vi "WM Create Wave Buffer with Phase Angle.vi"(2 "Buffer Info":T2 {"Paddle Height" format="%.2f"; "Water Depth" format="%.2f"}, 3 "Sine Paramaters":T1 {"Phase Angle (rad)" format="%.2f"; "Wave Height" format="%.2f"; "Period" format="%.2f"}) -> (0 "Output":dbl[](array[numeric]) format="%.2f", 1 "Buffer Size":i32)   [LabVIEW 2012]
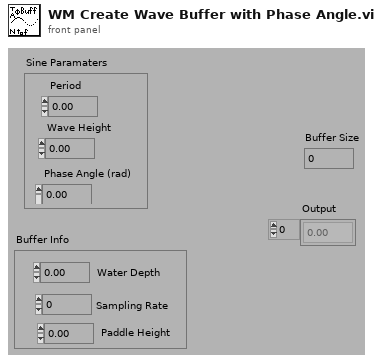
[diagram p1: front panel]
types:
  T1 = cluster{"Period":dbl, "Wave Height":dbl, "Phase Angle (rad)":dbl}
  T2 = cluster{"Sampling Rate":i32, "Water Depth":dbl, "Paddle Height":dbl}
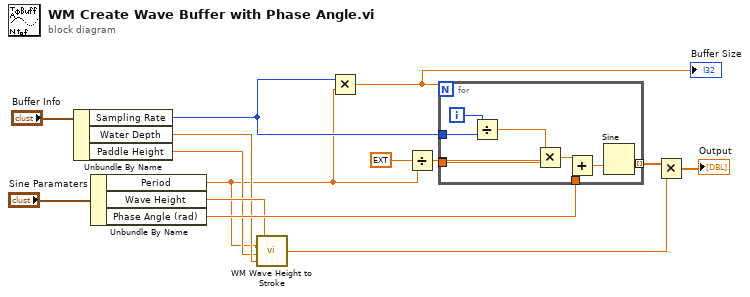
[diagram p0: block diagram]
diagram:
  n1 = Unbundle By Name("Buffer Info") -> ("Sampling Rate"=w5:i32, "Water Depth"=w3:dbl, "Paddle Height"=w2:dbl)
  n2 = Unbundle By Name("Sine Paramaters") -> ("Period"=w1:dbl, "Wave Height"=w7:dbl, "Phase Angle (rad)"=w9:dbl)
  n3 = call "WM Wave Height to Stroke.vi"("Water Depth (m)"=w3, "Flap Height (m)"=w2, "Wave Period (s)"=w1, "Wave Height (m)"=w7) -> ("Flap Amplitude (from x=0) (m)"=w6:dbl)
  n4 = Multiply(x=w5, y=w1) -> (x*y=w4:dbl)
  "Buffer Size" <- w4
  n5 = Divide(x=ext 6.283185307179586477, y=w1) -> (x/y=w14:ext)
  n6 = for {
    N: w4 -> [_]
    tunnel: [w21] -> _ mode=indexing
    tunnel: [w22] -> w12 mode=indexing
    tunnel: w14 -> [w21]
    tunnel: w5 -> [w19]
    tunnel: w9 -> [w16]
    i -> [w20]
    n7 = Divide(x=w20, y=w19) -> (x/y=w15:dbl)
    n8 = Multiply(x=w15, y=w21) -> (x*y=w18:ext)
    n9 = Add(x=w18, y=w16) -> (x+y=w17:ext)
    n10 = Sine(x=w17) -> (sin(x)=w22:ext)
  }
  n11 = Multiply(x=w12, y=w6) -> (x*y=→"Output":ext[])
